vi "Set Scan Engine Decimation.vi"(8 "error in":errorcluster, 10 "scan engine decimation":u16, 11 "scan engine custom device ref in":T1 format="%.0x") -> (0 "error out":errorcluster, 3 "scan engine custom device ref out":T1 format="%.0x")   [LabVIEW 2017, in "Scan Engine Scripting.lvlib"]
doc: "Writes the Scan Engine Decimation to the provided Scan Engine custom device reference."
uses:
  Scan Engine Scripting.lvlib
  <vilib>/NI Veristand/Custom Device API/Custom Device Item Ref.ctl
  Globals/Property Strings.vi
  <vilib>/NI Veristand/Custom Device API/Set Item Property (U32).vi
  Scan Engine Custom Device.lvlib
  <vilib>/NI Veristand/Custom Device API/Custom Device API.lvlib
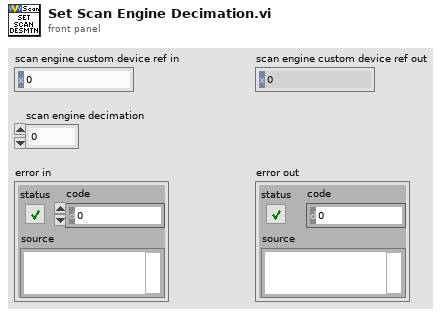
[diagram p1: front panel]
types:
  T1 = typedef "Custom Device API.lvlib/Custom Device Item Ref.ctl" = u64
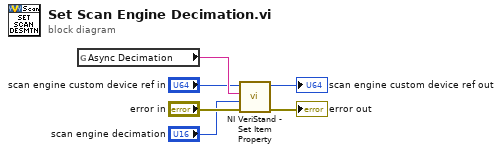
[diagram p0: block diagram]
diagram:
  n1 = global read "Property Strings.vi" "Async Decimation"() -> (w6:string)
  n2 = call-poly <vilib>:"NI VeriStand - Set Item Property.vi"("error in (no error)"="error in", "Value"="scan engine decimation", "Property Name"=w6, "Item Ref in"="scan engine custom device ref in") -> ("error out"=→"error out":errorcluster, "Item Ref out"=→"scan engine custom device ref out":T1)  [unwired: 5 in, 1 out]
